vi "RemoveCrates2.vi"(9 "From":i32, 10 "Qty":i32, 11 "StacksIn":cluster{"Crates":string[]}[](array[cluster])) -> (2 "CratesRemoved":string[](array[string]), 3 "StacksOut":cluster{"Crates":string[]}[](array[cluster]))   [LabVIEW 2020, in "2022_5.lvclass"]
uses:
  2022_5.lvclass
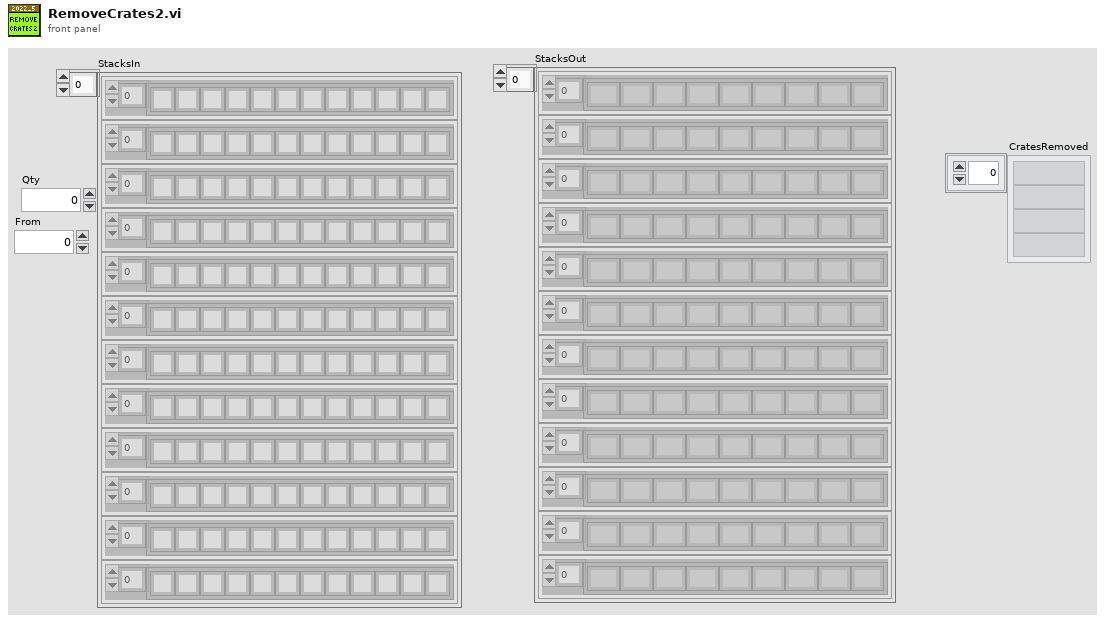
[diagram p1: front panel]
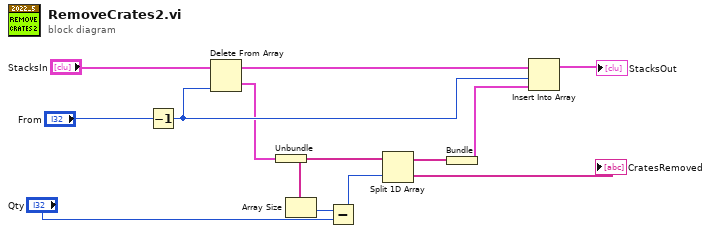
[diagram p0: block diagram]
diagram:
  n1 = Decrement(x="From") -> (x-1=w10:i32)
  n2 = Delete From Array(array="StacksIn", index=w10) -> (deleted portion=w8:cluster{"Crates":string[]}, array with subset deleted=w12:cluster{"Crates":string[]}[])  [unwired: 1 in]
  n3 = Unbundle(w8) -> ("Crates"=w7:string[])
  n4 = Array Size(array=w7) -> (size(s)=w6:i32)
  n5 = Subtract(x=w6, y="Qty") -> (x-y=w4:i32)
  n6 = Split 1D Array(array=w7, index=w4) -> (first subarray=w3:string[], second subarray=→"CratesRemoved":string[])
  n7 = Bundle(w3) -> (w2:cluster{string[]})  [unwired: 1 in]
  n8 = Insert Into Array(array=w12, index=w10, new element=w2) -> (→"StacksOut":cluster{"Crates":string[]}[])
